vi "Sent by myself QM.vi"(8 "error in (no error)":errorcluster, 10 "ProceedMessage":refnum<class "ProceedMessage.lvclass">, 11 "Autofocus in":refnum<class "Autofocus.lvclass">) -> (0 "error out":errorcluster, 1 "sent by myself?":bool, 2 "Message out":refnum<class "ProceedMessage.lvclass">, 3 "Autofocus out":refnum<class "Autofocus.lvclass">)   [LabVIEW 2012, in "Autofocus.lvclass"]
uses:
  Autofocus.lvclass
  <vilib>/Distrio/Murmex/ProceedMessage/ProceedMessage.lvclass
  <vilib>/Distrio/Murmex/Message/Message.lvclass
  <vilib>/Distrio/Murmex/Murmex/Murmex.lvclass
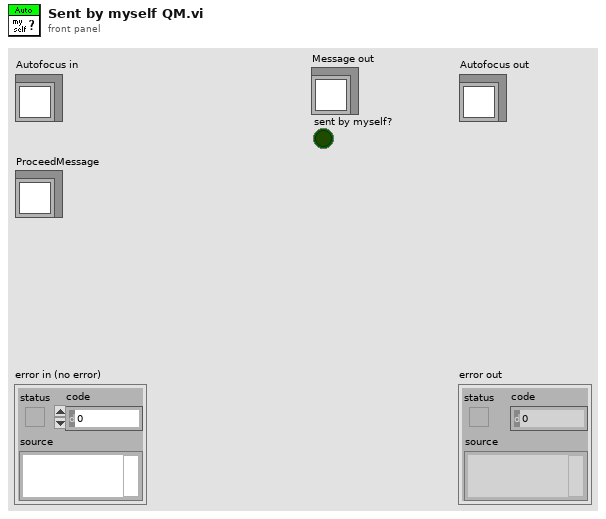
[diagram p1: front panel]
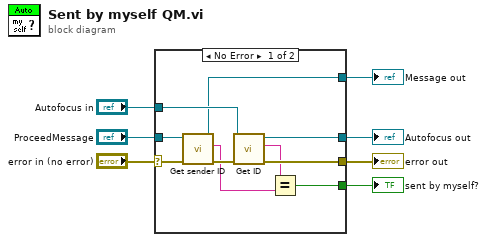
[diagram p0: block diagram]
diagram:
  n1 = case shown="No Error" "error in (no error)" {
    selector: "error in (no error)" -> [w15 w19]
    tunnel: [w14 w19] -> w6
    tunnel: [w12 w18] -> w4
    tunnel: "Autofocus in" -> [w13 w18]
    tunnel: "ProceedMessage" -> [w17 _]
    tunnel: [w11 _] -> w2
    tunnel: [w8 _] -> w1
    frame No Error {
      n2 = call <vilib>:"Get sender ID.vi"("error in (no error)"=w15, "Message in"=w17) -> ("error out"=w16:errorcluster, "sender"=w10:string, "Message out"=w11:refnum<class "ProceedMessage.lvclass">)  [unwired: 7 in]
      n3 = call <vilib>:"Get ID.vi"("error in (no error)"=w16, "Murmex in"=w13) -> ("error out"=w14:errorcluster, "component id"=w9:string, "Murmex out"=w12:refnum<class "Autofocus.lvclass">)  [unwired: 7 in]
      n4 = Equal?(x=w9, y=w10) -> (x = y?=w8:bool)
    }
    frame Error {
    }
  }
  "error out" <- w6
  "Autofocus out" <- w4
  "Message out" <- w2
  "sent by myself?" <- w1
